vi "Vision Tracking 2.vi"(0 "Image In":T2, 1 "Red or Hue Range (Color Threshold 1)":cluster{"Lower value":i32, "Upper value":i32}={"Lower value"=98, "Upper value"=153}, 2 "Green or Sat Range (Color Threshold 1)":cluster{"Lower value":i32, "Upper value":i32}={"Lower value"=222, "Upper value"=255}, 3 "Blue or Luma or Val or Inten Range (Color Threshold 1)":cluster{"Lower value":i32, "Upper value":i32}={"Lower value"=67, "Upper value"=140}, 7 "error in":errorcluster) -> (20 "Image Out":T2, 21 "Matches (Geometric Matching 1)":T1[](array[typedef]) {"Correlation Score" format="%.2f"; "Target Template Curve Score" format="%.2f"; "Template Target Curve Score" format="%.2f"; "Bounding Box"."y" format="%.2f"; "Bounding Box"."x" format="%.2f"; "Position"."y" format="%.2f"; "Position"."x" format="%.2f"; "Score" format="%.2f"; "Scale" format="%.2f"; "Angle" format="%.2f"; "Occlusion %" format="%.2f"}, 22 "Calibrated Matches (Geometric Matching 1)":T1[](array[typedef]) {"Correlation Score" format="%.2f"; "Target Template Curve Score" format="%.2f"; "Template Target Curve Score" format="%.2f"; "Bounding Box"."y" format="%.2f"; "Bounding Box"."x" format="%.2f"; "Position"."y" format="%.2f"; "Position"."x" format="%.2f"; "Score" format="%.2f"; "Scale" format="%.2f"; "Angle" format="%.2f"; "Occlusion %" format="%.2f"}, 23 "Number of Matches (Geometric Matching 1)":i32, 27 "error out":errorcluster)   [LabVIEW 2015]
uses:
  <vilib>/vision/Image Controls.llb/IMAQ Image.ctl
  <vilib>/vision/Pattern Matching.llb/IMAQ GM Match Report.ctl
  <vilib>/vision/Pattern Matching.llb/IMAQ Curve Parameters.ctl
  <vilib>/vision/Pattern Matching.llb/IMAQ Match Range Setting.ctl
  <vilib>/vision/NI_Vision_Development_Module.lvlib
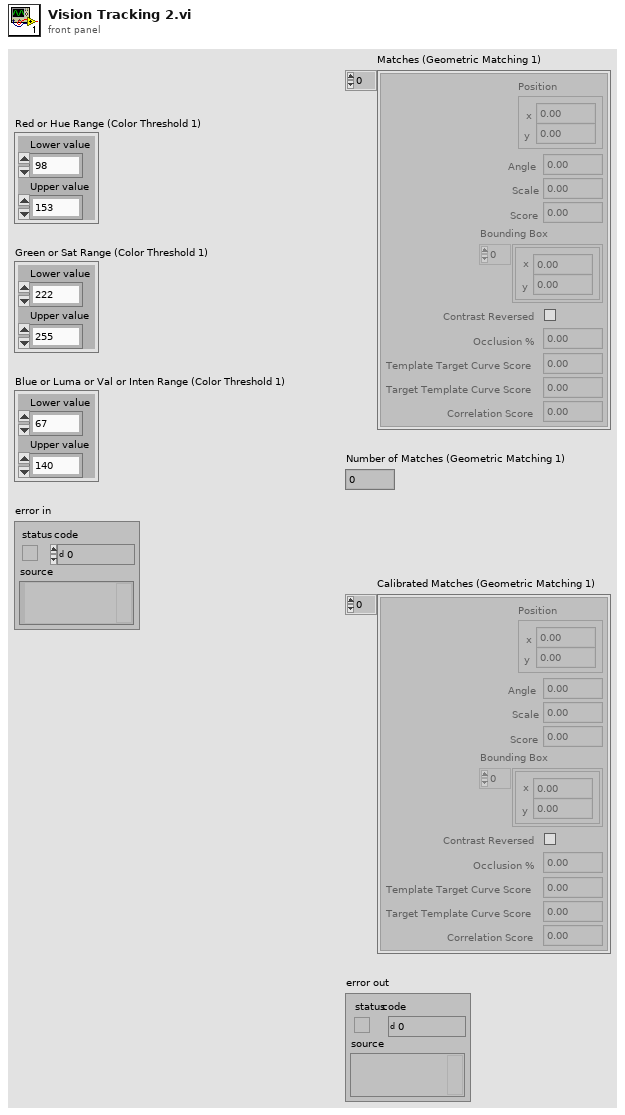
[diagram p1: front panel]
types:
  T1 = typedef "IMAQ GM Match Report.ctl" = cluster{"Position":cluster{"x":sgl, "y":sgl}, "Angle":sgl, "Scale":sgl, "Score":sgl, "Bounding Box":cluster{"x":sgl, "y":sgl}[], "Contrast Reversed":bool, "Occlusion %":sgl, "Template Target Curve Score":sgl, "Target Template Curve Score":sgl, "Correlation Score":sgl}
  T2 = typedef "IMAQ Image.ctl" = refnum<image>
  T3 = typedef "IMAQ Curve Parameters.ctl" = cluster{"Extraction Mode":u32, "Edge Threshold":i32, "Edge Filter Size":u32, "Min Length":i32, "Row Search Step Size":i32, "Col Search Step Size":i32, "Max Endpoint Gap":i32, "Closed":bool, "Subpixel":bool}
  T4 = typedef "IMAQ Match Range Setting.ctl" = cluster{"Match Constraints":u32, "Min":dbl, "Max":dbl}
  T5 = cluster{"Curve Parameters":T3, "Match Mode":cluster{"Rotation":bool, "Scale":bool, "Occlusion":bool, "Reserved":bool, "Reserved":bool, "Reserved":bool}, "Range Settings":T4[], "Number of Matches":i32, "Minimum Match Score":sgl, "SubPixel Accuracy":bool, "Adv. Geometric Match Options 2":cluster{"Setup Data Item":u16, "Item Value":dbl}[]}
  T6 = cluster{"Global Rectangle":i32[], "Contours":cluster{"ID":enum32{"External", "Internal"}, "Type":u32, "Coordinates":i32[]}[]}
  T7 = cluster{"histogram":u32[], "Minimal Value":sgl, "Maximal Value":sgl, "Starting Value":sgl, "Interval Width":sgl, "Mean Value":sgl, "Standard  Variation":sgl, "Area (pixels)":i32}
  T8 = typedef "Image Type" = u32
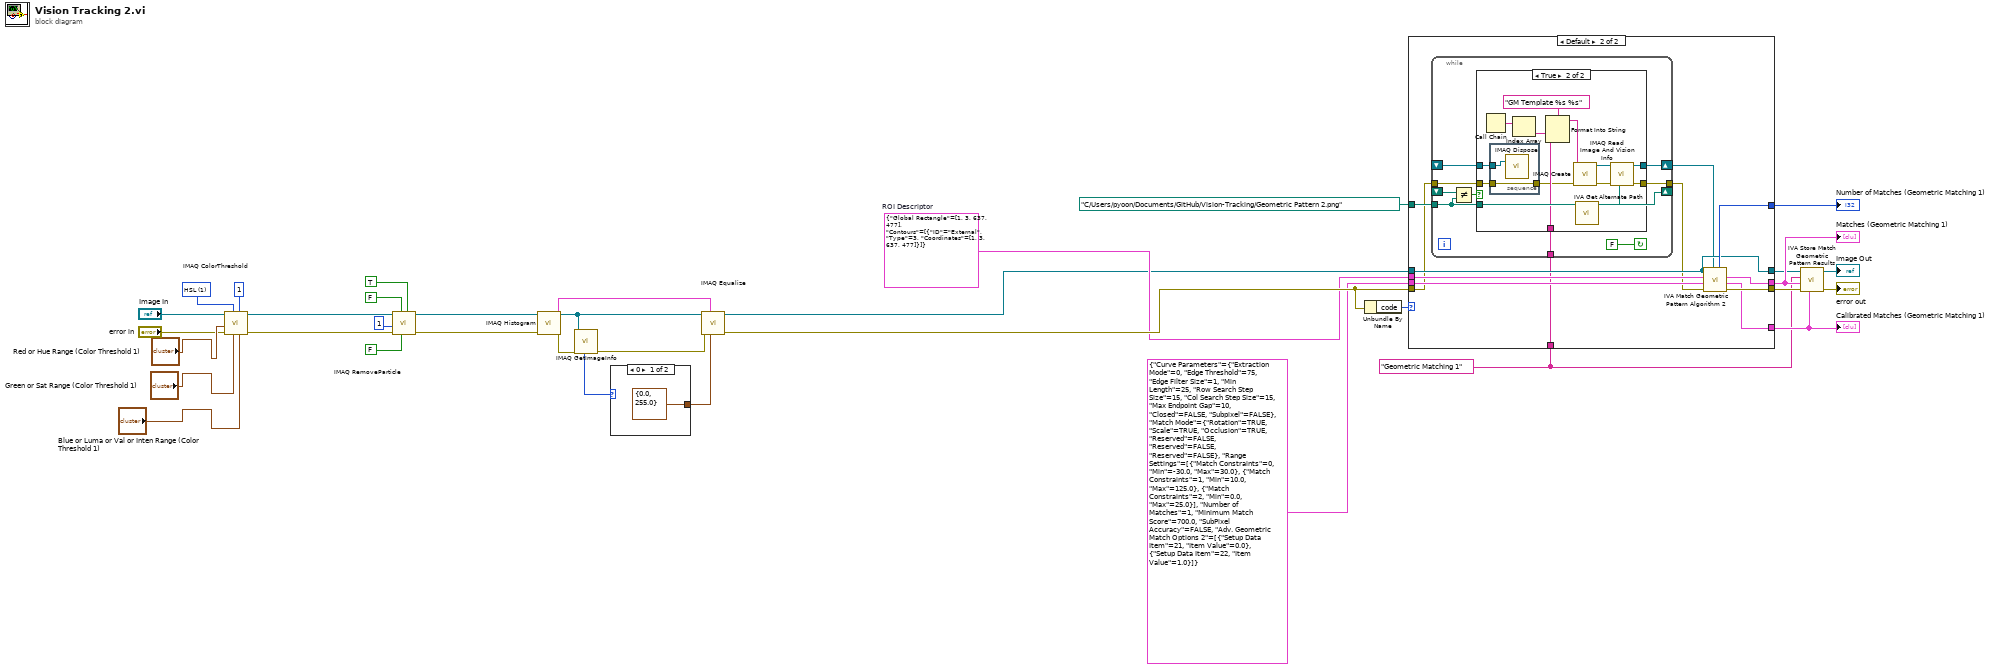
[diagram p0: block diagram]
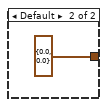
[diagram p4: hidden frame]
diagram:
  w1 = "Geometric Matching 1" ("Step Name")
  w12 = T6 {"Global Rectangle"=[1, 3, 637, 477], "Contours"=[{"ID"=enum."External", "Type"=3, "Coordinates"=[1, 3, 637, 477]}]}  # ROI Descriptor
  w33 = u16 1 items=["RGB", "HSL", "HSV", "HSI"] ("Color Mode")
  n1 = call "IMAQ ColorThreshold"("Blue or Luma or Val or Inten Range"="Blue or Luma or Val or Inten Range (Color Threshold 1)", "Replace Value"=1, "Green or Sat Range"="Green or Sat Range (Color Threshold 1)", "Color Mode"=w33, "error in (no error)"="error in", "Red or Hue Range"="Red or Hue Range (Color Threshold 1)", "Image Src"="Image In") -> ("error out"=w27:errorcluster, "Image Dst Out"=w22:T2)  [unwired: 1 in, 2 out]
  n2 = call "IMAQ RemoveParticle"("Connectivity 4/8 (8)"=TRUE, "Low Pass/High Pass (Low)"=FALSE, "Square/Hexa (Square)"=FALSE, "error in (no error)"=w27, "Number of Erosion"=1, "Image Src"=w22) -> ("error out"=w21:errorcluster, "Image Dst Out"=w17:T2)  [unwired: 1 in, 3 out]
  n3 = call "IMAQ Histogram"("error in (no error)"=w21, "Image"=w17) -> ("error out"=w16:errorcluster, "Histogram Report"=w19:T7)  [unwired: 3 in, 5 out]
  n4 = call "IMAQ GetImageInfo"("error in (no error)"=w16, "Image"=w17) -> ("error out"=w15:errorcluster, "Image Type"=w18:T8)  [unwired: 8 out]
  n5 = case shown="0" w18 {
    tunnel: [cluster{"Minimum":sgl, "Maximum":sgl} {"Minimum"=0.0, "Maximum"=255.0} ("Range") cluster{"Minimum":sgl, "Maximum":sgl} {"Minimum"=0.0, "Maximum"=0.0} ("Range")] -> w14
    frame 0 {
    }
    frame Default {
    }
  }
  n6 = call "IMAQ Equalize"("Range"=w14, "Histogram Report"=w19, "error in (no error)"=w15, "Image Src"=w17) -> ("error out"=w20:errorcluster, "Image Dst Out"=w11:T2)  [unwired: 2 in, 4 out]
  n7 = Unbundle By Name(w20) -> ("code"=w4:i32)
  n8 = case shown="Default" w4 {
    tunnel: path "C:/Users/pyoon/Documents/GitHub/Vision-Tracking/Geometric Pattern 2.png" ("Template File Path") -> [_ w42]
    tunnel: w20 -> [_ w41]
    tunnel: T5 {"Curve Parameters"={"Extraction Mode"=0, "Edge Threshold"=75, "Edge Filter Size"=1, "Min Length"=25, "Row Search Step Size"=15, "Col Search Step Size"=15, "Max Endpoint Gap"=10, "Closed"=FALSE, "Subpixel"=FALSE}, "Match Mode"={"Rotation"=TRUE, "Scale"=TRUE, "Occlusion"=TRUE, "Reserved"=FALSE, "Reserved"=FALSE, "Reserved"=FALSE}, "Range Settings"=[{"Match Constraints"=0, "Min"=-30.0, "Max"=30.0}, {"Match Constraints"=1, "Min"=10.0, "Max"=125.0}, {"Match Constraints"=2, "Min"=0.0, "Max"=25.0}], "Number of Matches"=1, "Minimum Match Score"=700.0, "SubPixel Accuracy"=FALSE, "Adv. Geometric Match Options 2"=[{"Setup Data Item"=21, "Item Value"=0.0}, {"Setup Data Item"=22, "Item Value"=1.0}]} ("Settings") -> [_ w49]
    tunnel: w12 -> [_ w48]
    tunnel: w11 -> [w37 w43]
    tunnel: [_ w47] -> w9
    tunnel: [_ w46] -> w7
    tunnel: [_ w45] -> w6
    tunnel: [_ w44] -> w5
    tunnel: [w37 w43] -> w3
    tunnel: w1 -> [_ w38]
    frame -1074396199, -1074396198 {
      # "Discard Coordinate System Error"
    }
    frame Default {
      n9 = while {
        shift-right: [w58] -> w39
        shift-left: _ -> [w57]
        tunnel: [w55] -> w40
        tunnel: w41 -> [w54]
        tunnel: w42 -> [w50]
        tunnel: w38 -> [w53]
        shift-right: [w50] -> _
        shift-left: _ -> [w52]
        stop <- FALSE continue-if-true
        n10 = Not Equal?(x=w52, y=w50) -> (x != y?=w51:bool)
        n11 = case shown="True" w51 {
          tunnel: [w60 w72] -> w58
          tunnel: w57 -> [w60 w64]
          tunnel: [w59 w69] -> w55
          tunnel: w54 -> [w59 w65]
          tunnel: w53 -> [_ w66]
          tunnel: w50 -> [_ w62]
          frame False {
          }
          frame True {
            n12 = Call Chain() -> (call chain=w68:string[])
            n13 = stacked-sequence {
              tunnel: w65 -> [w76]
              tunnel: w64 -> [w75]
              tunnel: [w76] -> w63
              frame #0 {
                n14 = call "IMAQ Dispose"("Image"=w75) -> ()  [unwired: 2 in, 4 out]
              }
            }
            n15 = Index Array(array=w68) -> (element=w67:string)  [unwired: 1 in]
            n16 = Format Into String(format string="GM Template %s %s" ("Image Name"), w67, w66) -> (resulting string=w74:string)  [unwired: 2 in, 1 out]
            n17 = call "IMAQ Create"("Image Name"=w74, "error in (no error)"=w63) -> ("New Image"=w71:T2, "error out"=w70:errorcluster)  [unwired: 2 in, 1 out]
            n18 = call <vilib>:"IVA Get Alternate Path.vi"("Path In"=w62) -> ("Path Out"=w61:path)  [unwired: 10 out]
            n19 = call "IMAQ Read Image And Vision Info"("File Path"=w61, "error in (no error)"=w70, "Image"=w71) -> ("error out"=w69:errorcluster, "Image Out"=w72:T2)  [unwired: 1 in, 6 out]
          }
        }
      }
      n20 = call <vilib>:"IVA Match Geometric Pattern Algorithm 2.vi"("Template"=w39, "error in (no error)"=w40, "Settings"=w49, "ROI Descriptor"=w48, "Image"=w43) -> ("error out"=w47:errorcluster, "Calibrated Matches"=w45:T1[], "Matches"=w46:T1[], "Number of Matches"=w44:i32)  [unwired: 1 in, 2 out]
    }
  }
  "Matches (Geometric Matching 1)" <- w7
  "Number of Matches (Geometric Matching 1)" <- w5
  "Calibrated Matches (Geometric Matching 1)" <- w6
  n21 = call <vilib>:"IVA Store Match Geometric Pattern Results.vi"("Calibrated Matches"=w6, "error in (no error)"=w9, "Matches"=w7, "Step Name"=w1, "Image in"=w3) -> ("error out"=→"error out":errorcluster, "Image dup"=→"Image Out":T2)  [unwired: 5 out]
